vi "UI.vi"(0 "reference in":refnum<class "GUI Script Editor.lvclass">, 5 "error in (no error)":errorcluster) -> (14 "reference out":refnum<class "GUI Script Editor.lvclass">, 19 "error out":errorcluster)   [LabVIEW 2019, in "GUI Script Editor.lvclass"]
uses:
  GUI Script Editor.lvclass
  D:/H4000/src/GUI_class/GUI.lvclass
  TypeDef/GUI Step.ctl
  GUI_class/GUI.lvclass/GUI.ctl
  ConfigJSON_class/ConfigJSON.lvclass
  TypeDef/Script.ctl
  TypeDef/Step.ctl
  TypeDef/Direction.ctl
  ConfigJSON_class/ConfigJSON.lvclass/ConfigJSON.ctl
  99d7901a-116f-403a-a3f6-606aa629af4a.vi
  e526d8fc-7282-4644-9dda-8724ecf4fc0a.vi
  GUI_class/Set Win State.vi
  GUI_class/protected/GetSheredData.vi
  GUI_class/GUI.lvclass
  45f5d260-08a4-4eac-ba28-dc2dcf1a59bc.vi
  ConfigInterface_class/ConfigInterface.lvclass
  2ddd2a0d-c32e-4038-aee9-799db4cb2551.vi
panel:
  in  "GUI Step":T1
  in  "create":bool
  in  "Add Step":bool
  out "XY Graph - Dark":cluster{"X":dbl[], "Y":dbl[]}[](graph) caption="Давление"
  in  "Delete step":bool
  out "Program name":string="Название"
  in  "Save As":bool
  in  "Open":bool
  in  "Save":bool
  in  "Steps":i32(listbox)
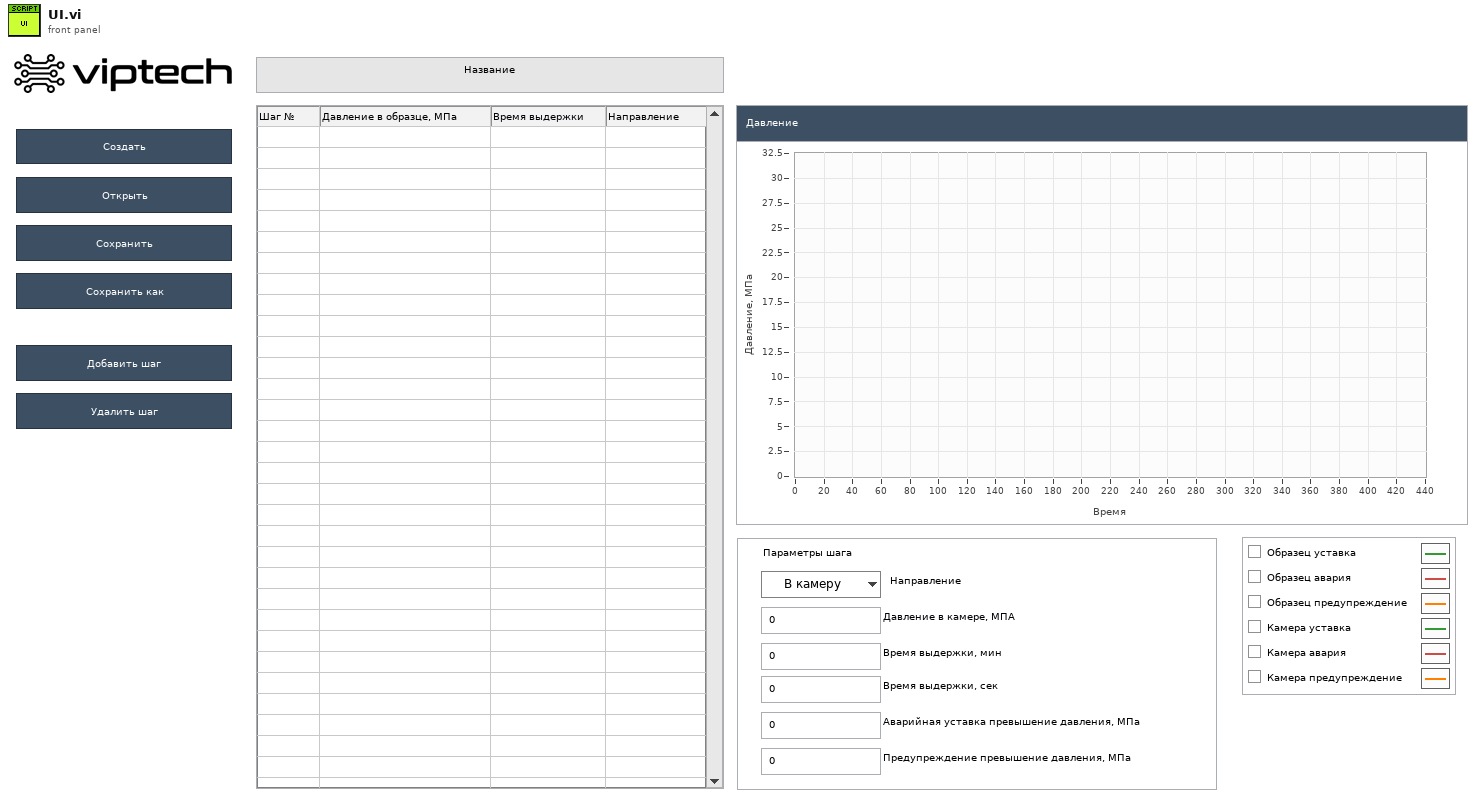
[diagram p1: front panel]
types:
  T1 = typedef "GUI Step.ctl" = cluster{"pressure MPa":dbl, "time min":dbl, "delta alarm MPa":dbl, "direction":enum16{"В камеру", "В образец"}, "delta warning MPa":dbl, "time sec":dbl}
  T2 = typedef "Script.ctl" = cluster{"Steps":T3[]}
  T3 = typedef "Step.ctl" = cluster{"Direction":T4, "Pressure MPa":dbl, "Time s":dbl, "Delta alarm MPa":dbl, "Delta warning MPa":dbl}
  T4 = typedef "Direction.ctl" = enum16{"Chamber", "DUT"}
  T5 = enum32{"Invalid", "Standard", "Closed", "Hidden", "Minimized", "Maximized"}
  T6 = enum32{"invalid app kind", "Development System", "Run Time System", "Student Edition", "Embedded LabVIEW", "Evaluation", "Custom"}
  T7 = cluster{"Core":cluster{"Current VI Reference":refnum<vi>, "Close Panel on Exit?":bool}, "Dir Scripts":path, "Curr Script":T2, "selected path":path, "Steps ref":refnum<vi>}
  T8 = cluster{"Current VI Reference":refnum<vi>, "Close Panel on Exit?":bool}
  T9 = typedef "GUI Paths.ctl" = cluster{"Dir Data":path, "Dir Setting":path, "SensorLib":path, "Dir Scripts":path}
  T10 = typedef "GUI Alarm customer settings.ctl" = cluster{"HIHI AI2":dbl, "HI AI2":dbl, "HIHI AI3":dbl, "HI AI3":dbl, "ENG0 OFF TIMEOUT":dbl, "ENG0 ON TIMEOUT":dbl, "HIHI AI7":dbl, "HI AI7":dbl, "HIHI AI6":dbl, "HI AI6":dbl, "HIHI AI5":dbl, "HI AI5":dbl}
  T11 = typedef "GUI Alarm developer settings.ctl" = cluster{"HIHI AI2":dbl, "HI AI2":dbl, "HIHI AI0":dbl, "HI AI0":dbl, "LOLO AI0":dbl, "LO AI0":dbl, "ENG2 OFF TIMEOUT":dbl, "ENG2 ON TIMEOUT":dbl, "HIHI AI3":dbl, "HI AI3":dbl, "HIHI AI1":dbl, "HI AI1":dbl, "LOLO AI1":dbl, "LO AI1":dbl, "ENG1 OFF TIMEOUT":dbl, "ENG1 ON TIMEOUT":dbl, "ENG0 OFF TIMEOUT":dbl, "ENG0 ON TIMEOUT":dbl, "LOLO AI8":dbl, "LO AI8":dbl, "LOLO AI9":dbl, "LO AI9":dbl, "LOLO AI5":dbl, "LO AI5":dbl, "Out Of Range HI":dbl, "Out Of Range LO":dbl}
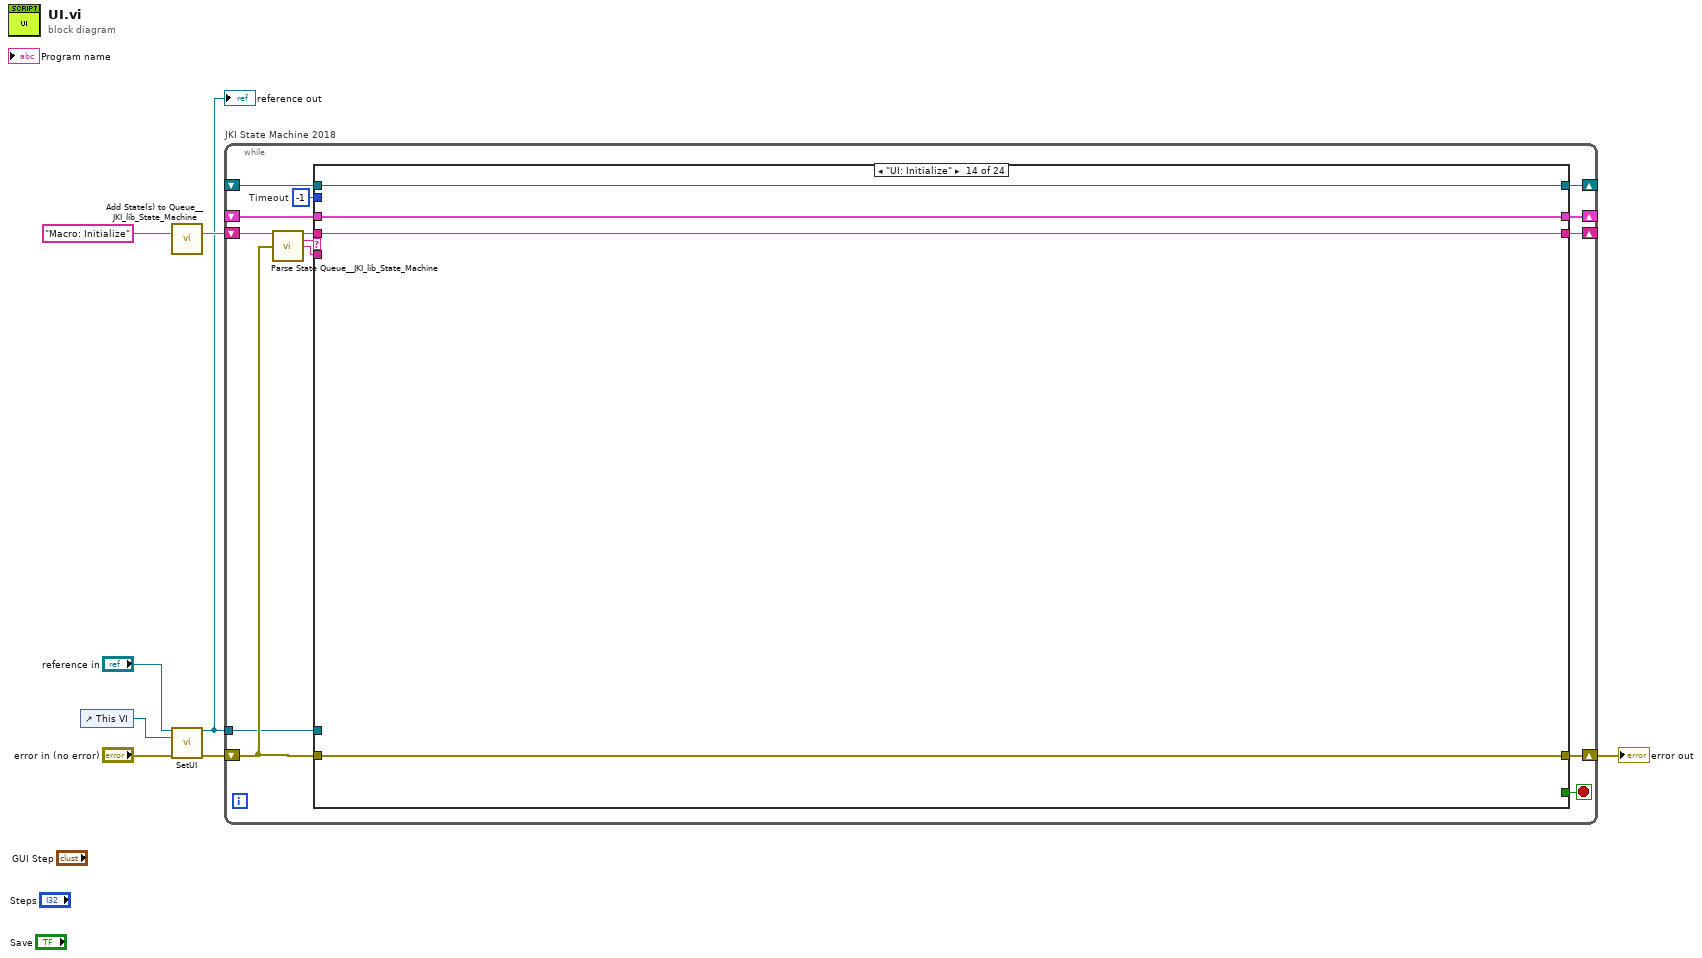
[diagram p0: block diagram]
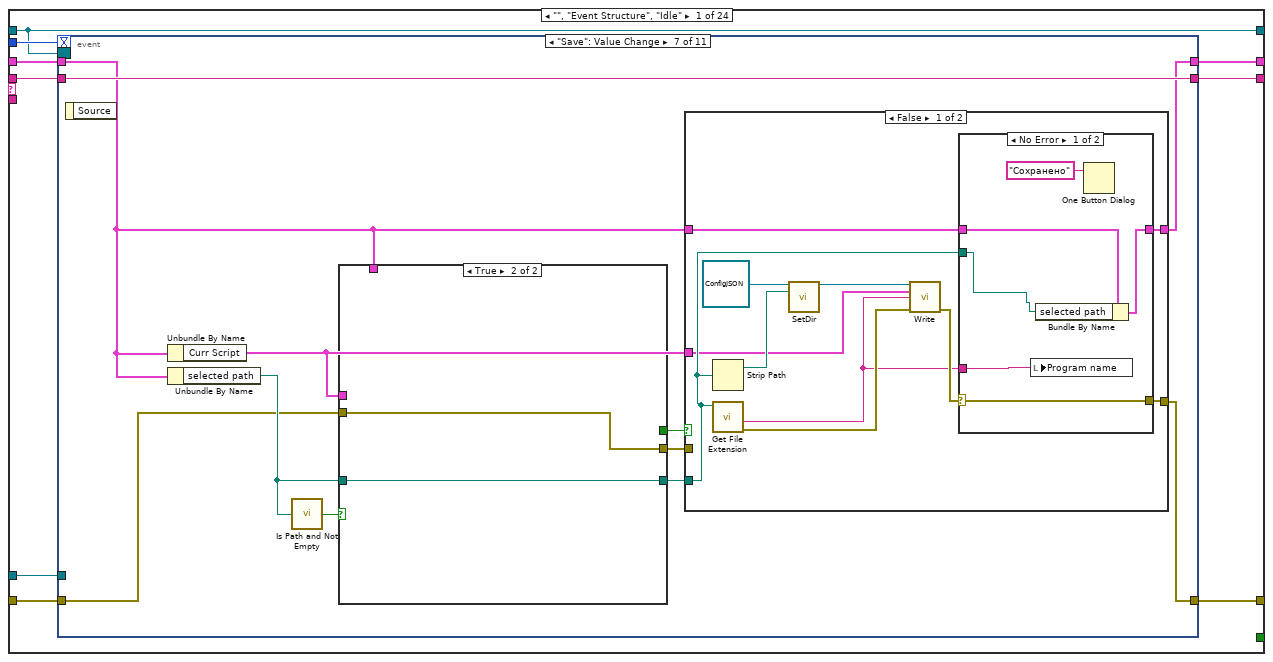
[diagram p2: hidden frame]
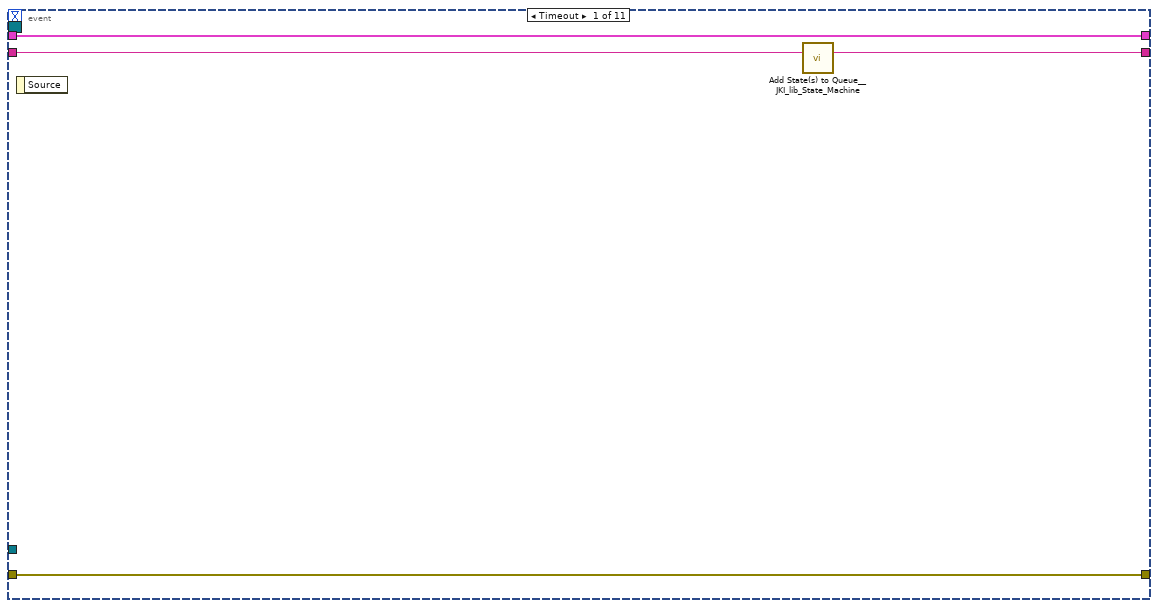
[diagram p3: hidden frame]
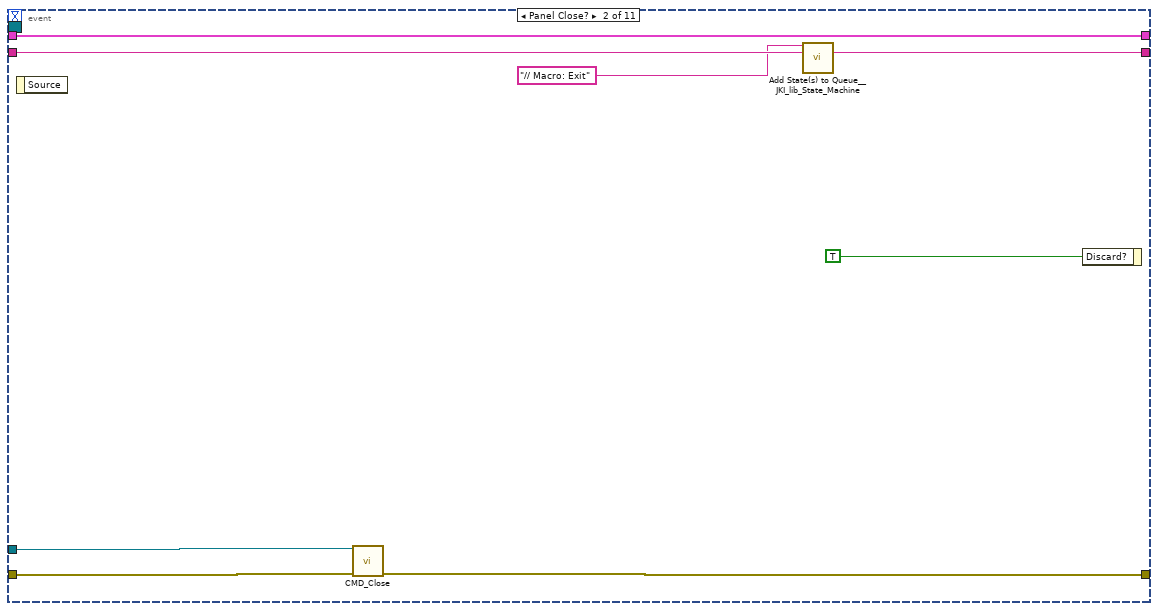
[diagram p4: hidden frame]
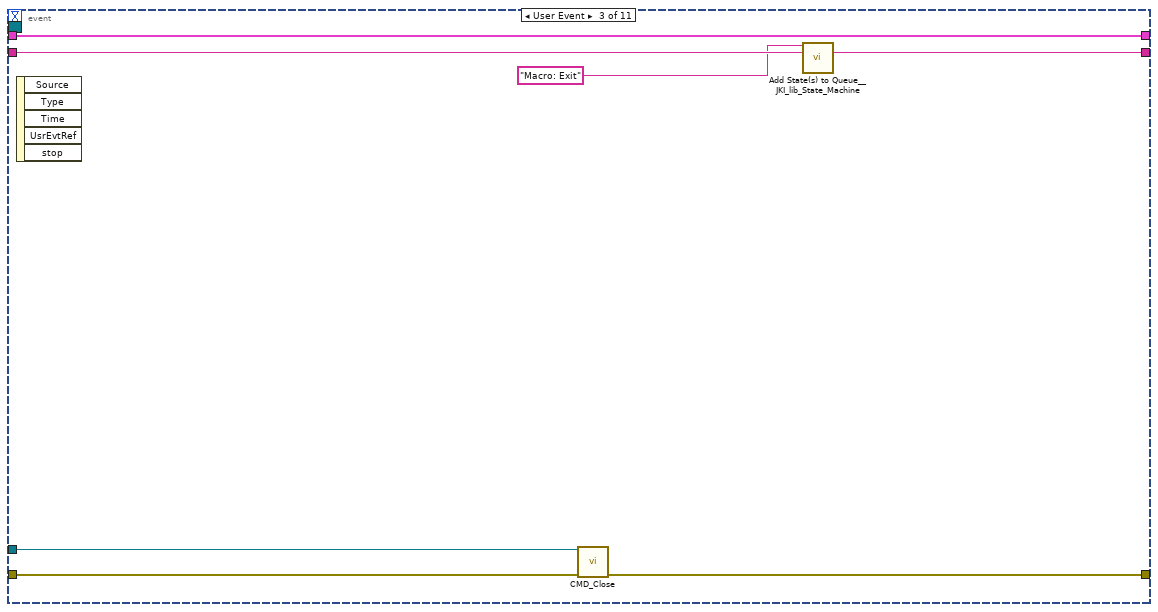
[diagram p5: hidden frame]
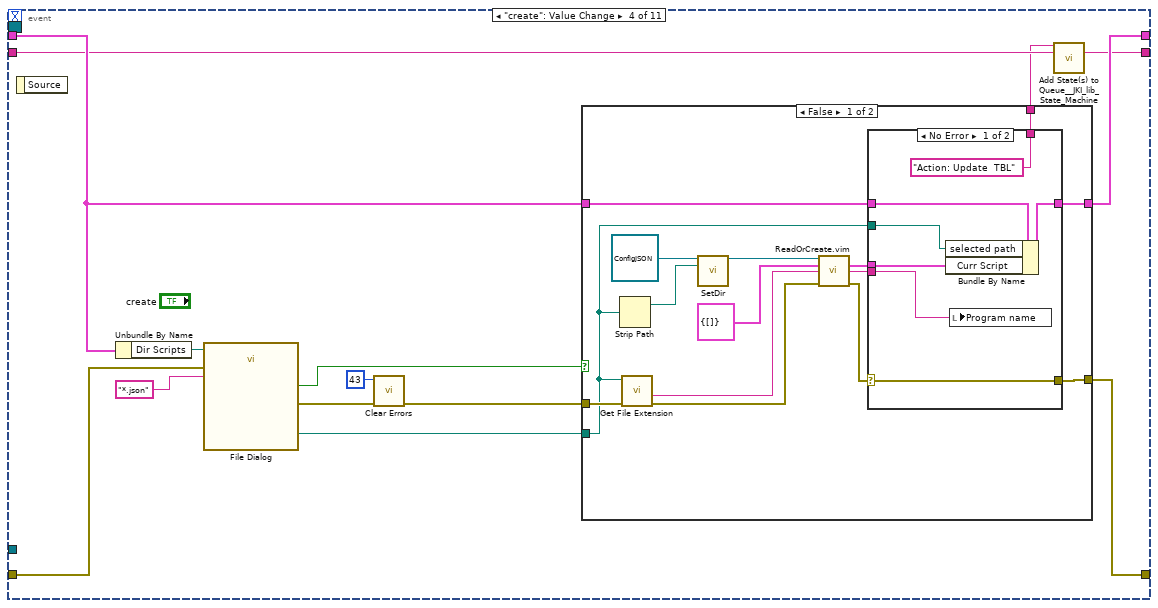
[diagram p6: hidden frame]
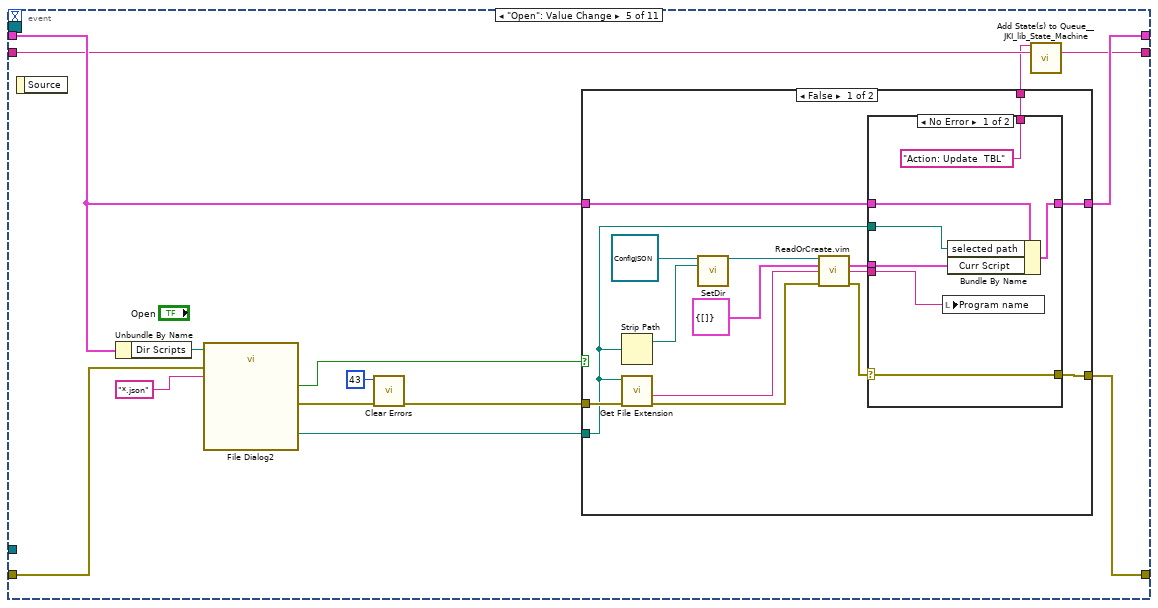
[diagram p9: hidden frame]
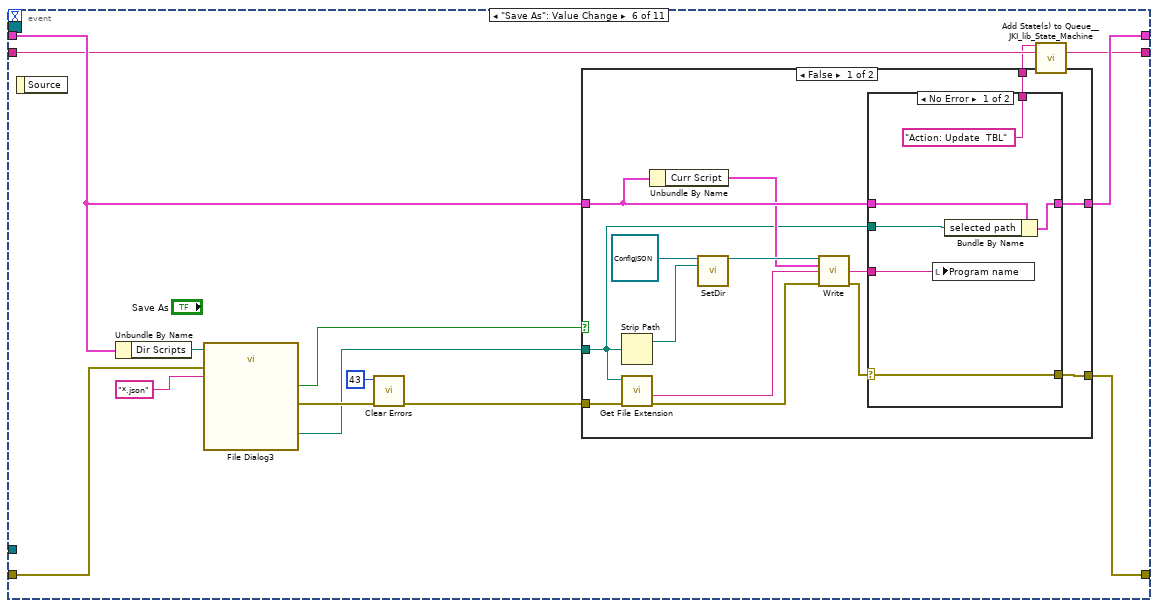
[diagram p12: hidden frame]
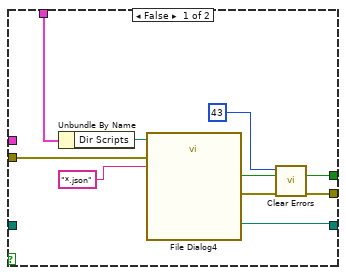
[diagram p17: hidden frame]
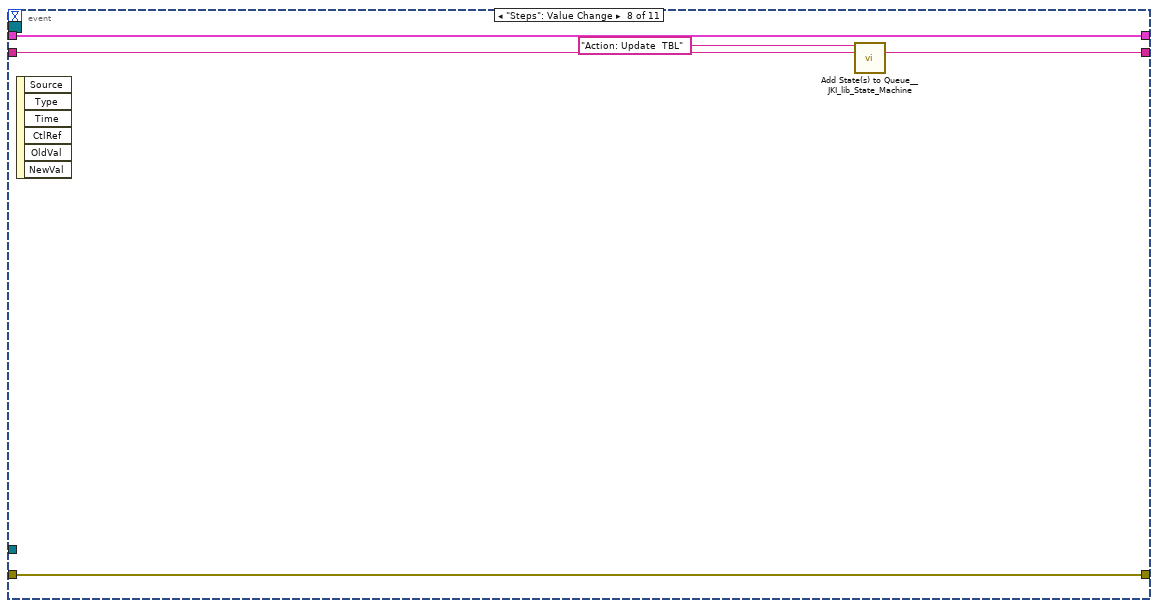
[diagram p18: hidden frame]
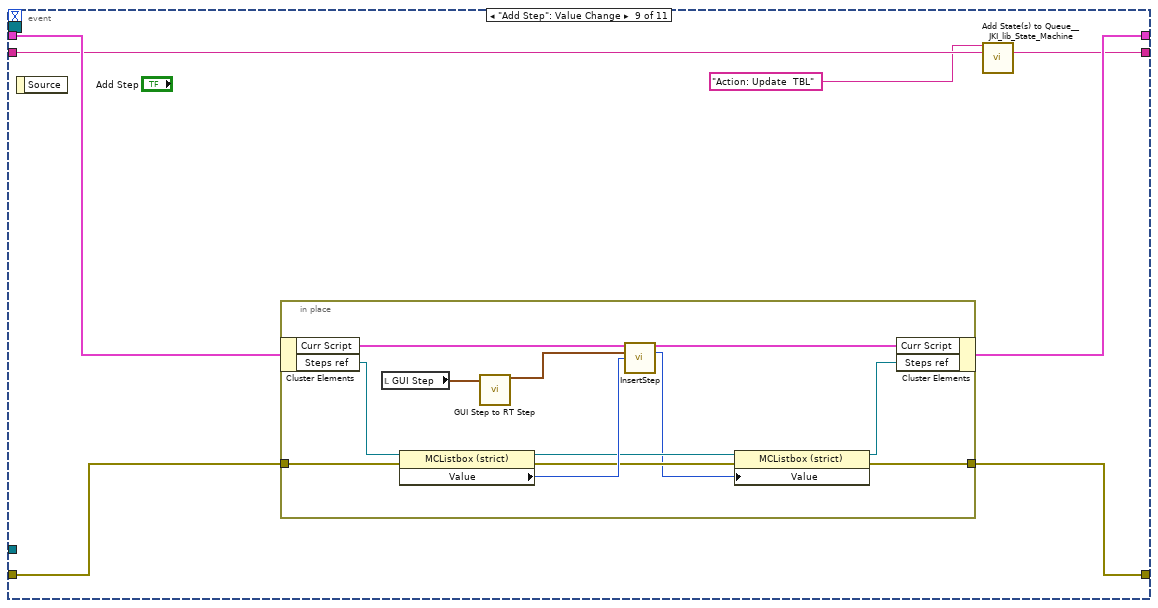
[diagram p19: hidden frame]
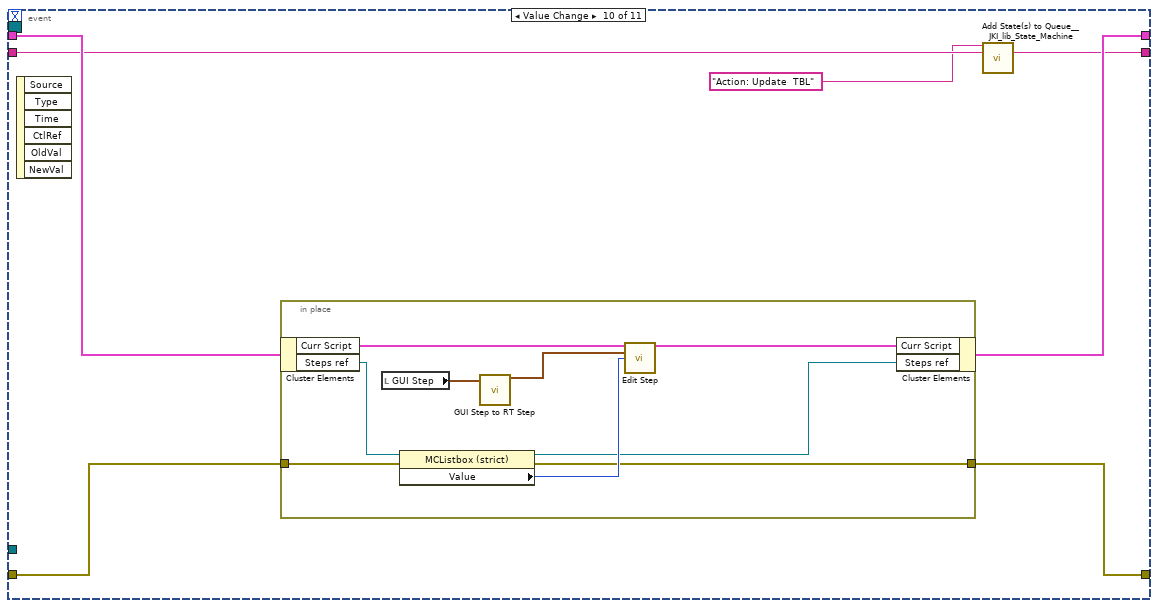
[diagram p20: hidden frame]
diagram:
  n1 = control-ref of="This VI"() -> (w3:refnum<vi>)
  n2 = call <vilib>:"Add State(s) to Queue__JKI_lib_State_Machine.vi"("State(s) in (\"\")"="Macro: Initialize") -> ("States Out"=w8:string)  [unwired: 14 in]
  n3 = call "SetUI.vi"("reference in"="reference in", "UI VI"=w3, "error in (no error)"="error in (no error)") -> ("reference out"=w1:refnum<class "GUI Script Editor.lvclass">, "error out"=w2:errorcluster)  [unwired: 11 in]
  "reference out" <- w1
  n4 = while "JKI State Machine 2018" {
    shift-right: [w15] -> _
    shift-left: _ -> [w14]
    shift-right: [w18] -> w6
    shift-left: w2 -> [w12]
    shift-right: [w17] -> _
    shift-left: w8 -> [w19]
    tunnel: w1 -> [w11]
    shift-right: [w10] -> _
    shift-left: _ -> [w9]
    stop <- w16 stop-if-true
    w13 = -1  # Timeout
    n5 = call <vilib>:"Parse State Queue__JKI_lib_State_Machine.vi"("State Queue"=w19, "Error In (no error)"=w12) -> ("Remaining States"=w21:string, "Current State"=w22:string, "Arguments"=w20:string)  [unwired: 11 in]
    n6 = case shown="\"UI: Initialize\"" w22 {
      selector: w22 -> [_ _ w275 _ _ _ _ _ _ _ _ _ _ _ _ _ _ _ _ _ _ _ _ _]
      tunnel: w21 -> [w31 w273 w279 w299 w306 w312 w317 w328 w335 w340 w347 w353 w358 w362 w369 w381 w451 w457 w463 w475 w479 w488 w512 w539]
      tunnel: w20 -> [_ _ _ _ _ _ _ _ _ _ _ _ _ _ w364 w375 _ _ _ _ _ _ _ _]
      tunnel: w14 -> [w29 w270 w277 w292 w303 w310 w314 _ w330 w337 w346 w351 w355 w361 w367 w377 w448 w454 w460 w472 w477 w483 w508 w538]
      tunnel: [w28 w271 w281 w296 errorcluster {"status"=FALSE, "code"=0, "source"=""} ("error out") w309 w315 w321 w331 w338 w344 w348 w356 w360 w365 w378 w449 w455 w461 w473 w478 w482 w507 w534] -> w18
      tunnel: w12 -> [w27 w271 w280 w296 w302 w309 w315 w323 w332 w338 w343 w349 w356 w360 w366 w379 w449 w455 w461 w473 w478 w481 w509 w535]
      tunnel: [w30 w272 w278 w298 w305 w311 w316 w328 w334 w339 w347 w352 w357 w362 w368 w380 w450 w456 w462 w474 w479 w488 w512 w539] -> w17
      tunnel: [_ _ _ _ _ TRUE _ _ _ _ _ _ _ _ _ _ _ _ _ _ _ _ _ _] -> w16
      tunnel: [w26 w270 w277 w297 w303 w310 w314 w327 w330 w337 w346 w351 w355 w361 w367 w377 w448 w454 w460 w472 w477 w486 w508 w538] -> w15
      tunnel: w13 -> [w25 _ _ _ _ _ _ _ _ _ _ _ _ _ _ _ _ _ _ _ _ _ _ _]
      tunnel: w11 -> [w24 _ _ _ _ _ _ _ _ _ w342 _ _ _ _ _ _ _ _ _ _ w485 w510 _]
      tunnel: [w23 w269 w274 w286 w300 w307 w313 w325 w329 w336 w345 w350 w354 w359 w363 w374 w447 w452 w458 w465 w476 w487 w511 w540] -> w10
      tunnel: w9 -> [w23 w269 w274 w286 w300 w307 w313 w325 w329 w336 _ w350 w354 w359 w363 w374 w447 w452 w458 w465 w476 w487 w511 w540]
      frame "", "Event Structure", "Idle" {
        n7 = event shown="[6] \"Save\": Value Change" {
          selector: w23 -> [_ _ _ _ _ _ _ _ _ _ _]
          dyn-events: _ -> [_ _ _ _ _ _ _ _ _ _ _]
          timeout: w25 -> [_ _ _ _ _ _ _ _ _ _ _]
          tunnel: w31 -> [w35 w43 w50 w52 w92 w132 w179 w213 w218 w237 w253]
          tunnel: [w34 w42 w49 w53 w93 w133 w179 w214 w219 w238 w254] -> w30
          tunnel: w29 -> [w32 w41 w48 w55 w95 w135 w171 w215 w223 w242 w258]
          tunnel: [w33 w36 w44 w57 w97 w137 w178 w216 w220 w239 w255] -> w28
          tunnel: w27 -> [w33 w37 w45 w63 w103 w143 w173 w216 w221 w240 w256]
          tunnel: [w32 w41 w48 w54 w94 w134 w177 w215 w222 w241 w257] -> w26
          tunnel: w24 -> [_ w38 w46 _ _ _ _ _ _ _ _]
          event Timeout {
            n8 = event-data() -> ()  [unwired: 1 in, 1 out]
            n9 = call <vilib>:"Add State(s) to Queue__JKI_lib_State_Machine.vi"("State(s) in (\"\")"=w35) -> ("States Out"=w34:string)  [unwired: 14 in]
          }
          event Panel Close? {
            n10 = event-data() -> ()  [unwired: 1 in, 1 out]
            n11 = call "CMD_Close.vi"("reference in"=w38, "error in (no error)"=w37) -> ("error out"=w36:errorcluster)  [unwired: 12 in, 1 out]
            n12 = call <vilib>:"Add State(s) to Queue__JKI_lib_State_Machine.vi"("State(s) in Front (\"\")"="// Macro: Exit", "State(s) in (\"\")"=w43) -> ("States Out"=w42:string)  [unwired: 13 in]
            n13 = event-data("Discard?"=TRUE) -> ()  [unwired: 1 in, 1 out]
          }
          event User Event {
            n14 = event-data() -> ()  [unwired: 1 in, 5 out]
            n15 = call "CMD_Close.vi"("reference in"=w46, "error in (no error)"=w45) -> ("error out"=w44:errorcluster)  [unwired: 12 in, 1 out]
            n16 = call <vilib>:"Add State(s) to Queue__JKI_lib_State_Machine.vi"("State(s) in Front (\"\")"="Macro: Exit", "State(s) in (\"\")"=w50) -> ("States Out"=w49:string)  [unwired: 13 in]
          }
          event "create": Value Change {
            n17 = event-data() -> ()  [unwired: 1 in, 1 out]
            n18 = Unbundle By Name(w55) -> ("Dir Scripts"=w64:path)
            n19 = call "File Dialog"("start path"=w64, "error in"=w63, "pattern (all files)"="*.json") -> ("selected path"=w56:path, "cancelled"=w58:bool, "error out"=w60:errorcluster)  [unwired: 9 in, 1 out]
            n20 = call <vilib>:"Clear Errors.vi"("error in (no error)"=w60, "specific error code to clear (0: all)"=43) -> ("error out"=w59:errorcluster)  [unwired: 4 in, 1 out]
            n21 = case shown="False" w58 {
              tunnel: w59 -> [w76 w90]
              tunnel: [w71 w90] -> w57
              tunnel: w56 -> [w66 _]
              tunnel: w55 -> [w70 w89]
              tunnel: [w69 w89] -> w54
              tunnel: [w65 _] -> w51
              frame False {
                n22 = Strip Path(path=w66) -> (stripped path=w77:path)  [unwired: 1 out]
                n23 = call <vilib>:"Get File Extension.vi"("error in (no error)"=w76, "file"=w66) -> ("error out"=w73:errorcluster, "filename without extension"=w75:string)  [unwired: 5 in, 3 out]
                n24 = call "SetDir.vi"("reference in"=refnum<class "ConfigJSON.lvclass"> refnum ("ConfigJSON"), "Config Dir"=w77) -> ("JSON"=w78:refnum<class "ConfigJSON.lvclass">)  [unwired: 13 in]
                n25 = call "ReadOrCreate.vim"("reference in"=w78, "Type and Defaults"=T2 {"Steps"=[]} ("Script"), "Name"=w75, "error in (no error)"=w73) -> ("Data"=w68:T2, "Name dub"=w67:string, "error out"=w72:errorcluster)  [unwired: 7 in, 2 out]
                n26 = case shown="No Error" w72 {
                  selector: w72 -> [w83 w88]
                  tunnel: [w83 w88] -> w71
                  tunnel: w70 -> [w86 w87]
                  tunnel: [w85 w87] -> w69
                  tunnel: w68 -> [w84 _]
                  tunnel: w67 -> [w82 _]
                  tunnel: w66 -> [w81 _]
                  tunnel: ["Action: Update  TBL" ("State(s) in Front (\"\")") _] -> w65
                  frame No Error {
                    n27 = Bundle By Name(cluster=w86, "selected path"=w81, "Curr Script"=w84) -> (w85:T7)
                    n28 = local write "Program name"(w82) -> ()
                  }
                  frame Error {
                  }
                }
              }
              frame True {
              }
            }
            n29 = call <vilib>:"Add State(s) to Queue__JKI_lib_State_Machine.vi"("State(s) in Front (\"\")"=w51, "State(s) in (\"\")"=w52) -> ("States Out"=w53:string)  [unwired: 13 in]
          }
          event "Open": Value Change {
            n30 = event-data() -> ()  [unwired: 1 in, 1 out]
            n31 = Unbundle By Name(w95) -> ("Dir Scripts"=w104:path)
            n32 = call "File Dialog2"("start path"=w104, "error in"=w103, "pattern (all files)"="*.json") -> ("selected path"=w96:path, "cancelled"=w98:bool, "error out"=w100:errorcluster)  [unwired: 9 in, 1 out]
            n33 = call <vilib>:"Clear Errors.vi"("error in (no error)"=w100, "specific error code to clear (0: all)"=43) -> ("error out"=w99:errorcluster)  [unwired: 4 in, 1 out]
            n34 = case shown="False" w98 {
              tunnel: w99 -> [w116 w130]
              tunnel: [w111 w130] -> w97
              tunnel: w96 -> [w106 _]
              tunnel: w95 -> [w110 w129]
              tunnel: [w109 w129] -> w94
              tunnel: [w105 _] -> w91
              frame False {
                n35 = Strip Path(path=w106) -> (stripped path=w117:path)  [unwired: 1 out]
                n36 = call <vilib>:"Get File Extension.vi"("error in (no error)"=w116, "file"=w106) -> ("error out"=w113:errorcluster, "filename without extension"=w115:string)  [unwired: 5 in, 3 out]
                n37 = call "SetDir.vi"("reference in"=refnum<class "ConfigJSON.lvclass"> refnum ("ConfigJSON"), "Config Dir"=w117) -> ("JSON"=w118:refnum<class "ConfigJSON.lvclass">)  [unwired: 13 in]
                n38 = call "ReadOrCreate.vim"("reference in"=w118, "Type and Defaults"=T2 {"Steps"=[]} ("Script"), "Name"=w115, "error in (no error)"=w113) -> ("Data"=w108:T2, "Name dub"=w107:string, "error out"=w112:errorcluster)  [unwired: 7 in, 2 out]
                n39 = case shown="No Error" w112 {
                  selector: w112 -> [w123 w128]
                  tunnel: [w123 w128] -> w111
                  tunnel: w110 -> [w126 w127]
                  tunnel: [w125 w127] -> w109
                  tunnel: w108 -> [w124 _]
                  tunnel: w107 -> [w122 _]
                  tunnel: w106 -> [w121 _]
                  tunnel: ["Action: Update  TBL" ("State(s) in Front (\"\")") _] -> w105
                  frame No Error {
                    n40 = local write "Program name"(w122) -> ()
                    n41 = Bundle By Name(cluster=w126, "selected path"=w121, "Curr Script"=w124) -> (w125:T7)
                  }
                  frame Error {
                  }
                }
              }
              frame True {
              }
            }
            n42 = call <vilib>:"Add State(s) to Queue__JKI_lib_State_Machine.vi"("State(s) in Front (\"\")"=w91, "State(s) in (\"\")"=w92) -> ("States Out"=w93:string)  [unwired: 13 in]
          }
          event "Save As": Value Change {
            n43 = event-data() -> ()  [unwired: 1 in, 1 out]
            n44 = Unbundle By Name(w135) -> ("Dir Scripts"=w144:path)
            n45 = call "File Dialog3"("start path"=w144, "error in"=w143, "pattern (all files)"="*.json") -> ("selected path"=w136:path, "cancelled"=w138:bool, "error out"=w140:errorcluster)  [unwired: 9 in, 1 out]
            n46 = call <vilib>:"Clear Errors.vi"("error in (no error)"=w140, "specific error code to clear (0: all)"=43) -> ("error out"=w139:errorcluster)  [unwired: 4 in, 1 out]
            n47 = case shown="False" w138 {
              tunnel: w139 -> [w155 w168]
              tunnel: [w151 w168] -> w137
              tunnel: w136 -> [w146 _]
              tunnel: w135 -> [w148 w167]
              tunnel: [w150 w167] -> w134
              tunnel: [w145 _] -> w131
              frame False {
                n48 = Strip Path(path=w146) -> (stripped path=w156:path)  [unwired: 1 out]
                n49 = call <vilib>:"Get File Extension.vi"("error in (no error)"=w155, "file"=w146) -> ("error out"=w153:errorcluster, "filename without extension"=w154:string)  [unwired: 5 in, 3 out]
                n50 = Unbundle By Name(w148) -> ("Curr Script"=w147:T2)
                n51 = call "SetDir.vi"("reference in"=refnum<class "ConfigJSON.lvclass"> refnum ("ConfigJSON"), "Config Dir"=w156) -> ("JSON"=w157:refnum<class "ConfigJSON.lvclass">)  [unwired: 13 in]
                n52 = call-dynamic "Write.vi"("reference in"=w157, "Data"=w147, "Name"=w154, "error in (no error)"=w153) -> ("Name dub"=w149:string, "error out"=w152:errorcluster)  [unwired: 8 in, 2 out]
                n53 = case shown="No Error" w152 {
                  selector: w152 -> [w162 w166]
                  tunnel: [w162 w166] -> w151
                  tunnel: w148 -> [w164 w165]
                  tunnel: [w163 w165] -> w150
                  tunnel: w149 -> [w161 _]
                  tunnel: w146 -> [w160 _]
                  tunnel: ["Action: Update  TBL" ("State(s) in Front (\"\")") _] -> w145
                  frame No Error {
                    n54 = local write "Program name"(w161) -> ()
                    n55 = Bundle By Name(cluster=w164, "selected path"=w160) -> (w163:T7)
                  }
                  frame Error {
                  }
                }
              }
              frame True {
              }
            }
            n56 = call <vilib>:"Add State(s) to Queue__JKI_lib_State_Machine.vi"("State(s) in Front (\"\")"=w131, "State(s) in (\"\")"=w132) -> ("States Out"=w133:string)  [unwired: 13 in]
          }
          event "Save": Value Change {
            n57 = event-data() -> ()  [unwired: 1 in, 1 out]
            n58 = Unbundle By Name(w171) -> ("Curr Script"=w172:T2)
            n59 = Unbundle By Name(w171) -> ("selected path"=w174:path)
            n60 = call <vilib>:"Is Path and Not Empty.vi"("path"=w174) -> ("Is Path and Not Empty?"=w176:bool)  [unwired: 4 in]
            n61 = case shown="True" w176 {
              tunnel: [w206 w211] -> w175
              tunnel: w174 -> [_ w211]
              tunnel: w173 -> [w207 w210]
              tunnel: w172 -> [_ _]
              tunnel: w171 -> [w205 _]
              tunnel: [w204 _] -> w170
              tunnel: [w201 w210] -> w169
              frame False {
                n62 = Unbundle By Name(w205) -> ("Dir Scripts"=w209:path)
                n63 = call "File Dialog4"("start path"=w209, "error in"=w207, "pattern (all files)"="*.json") -> ("selected path"=w206:path, "cancelled"=w204:bool, "error out"=w202:errorcluster)  [unwired: 9 in, 1 out]
                n64 = call <vilib>:"Clear Errors.vi"("error in (no error)"=w202, "specific error code to clear (0: all)"=43) -> ("error out"=w201:errorcluster)  [unwired: 4 in, 1 out]
              }
              frame True {
              }
            }
            n65 = case shown="False" w170 {
              tunnel: [w190 w199] -> w178
              tunnel: [w189 w200] -> w177
              tunnel: w175 -> [w183 _]
              tunnel: w172 -> [w182 _]
              tunnel: w171 -> [w181 w200]
              tunnel: w169 -> [_ w199]
              frame False {
                n66 = Strip Path(path=w183) -> (stripped path=w186:path)  [unwired: 1 out]
                n67 = call <vilib>:"Get File Extension.vi"("file"=w183) -> ("error out"=w185:errorcluster, "filename without extension"=w180:string)  [unwired: 6 in, 3 out]
                n68 = call "SetDir.vi"("reference in"=refnum<class "ConfigJSON.lvclass"> refnum ("ConfigJSON"), "Config Dir"=w186) -> ("JSON"=w187:refnum<class "ConfigJSON.lvclass">)  [unwired: 13 in]
                n69 = call-dynamic "Write.vi"("reference in"=w187, "Data"=w182, "Name"=w180, "error in (no error)"=w185) -> ("error out"=w184:errorcluster)  [unwired: 8 in, 3 out]
                n70 = case shown="No Error" w184 {
                  selector: w184 -> [w196 w198]
                  tunnel: [w196 w198] -> w190
                  tunnel: w181 -> [w192 w197]
                  tunnel: [w191 w197] -> w189
                  tunnel: w183 -> [w193 _]
                  tunnel: w180 -> [w194 _]
                  frame No Error {
                    n71 = local write "Program name"(w194) -> ()
                    n72 = Bundle By Name(cluster=w192, "selected path"=w193) -> (w191:T7)
                    n73 = One Button Dialog(message="Сохранено") -> ()  [unwired: 1 in, 1 out]
                  }
                  frame Error {
                  }
                }
              }
              frame True {
              }
            }
          }
          event "Steps": Value Change {
            n74 = event-data() -> ()  [unwired: 1 in, 6 out]
            n75 = call <vilib>:"Add State(s) to Queue__JKI_lib_State_Machine.vi"("State(s) in Front (\"\")"="Action: Update  TBL" ("State(s) in Front (\"\")"), "State(s) in (\"\")"=w213) -> ("States Out"=w214:string)  [unwired: 13 in]
          }
          event "Add Step": Value Change {
            n76 = event-data() -> ()  [unwired: 1 in, 1 out]
            n77 = in-place {
              in-place-border: w221 -> [w229]
              in-place-border: [w225] -> w220
              n78 = in-place-cluster #1(w223) -> ("Curr Script"=w235:T2, "Steps ref"=w232:refnum<vi>)
              n79 = local read "GUI Step"() -> (w231:T1)
              n80 = property class="MCListbox (strict)"(reference=w232, error in=w229) -> (reference out=w227:refnum<vi>, error out=w228:errorcluster, "Value"=w233:i32)
              n81 = call "GUI Step to RT Step.vi"("GUI Step"=w231) -> ("STEP"=w230:T3)  [unwired: 14 in]
              n82 = call "InsertStep.vi"("Script in"=w235, "new element/subarray"=w230, "index in"=w233) -> ("Script out"=w234:T2, "index out"=w224:i32)  [unwired: 11 in]
              n83 = property class="MCListbox (strict)"(reference=w227, error in=w228, "Value"=w224) -> (reference out=w226:refnum<vi>, error out=w225:errorcluster)
              n84 = in-place-cluster #1("Curr Script"=w234, "Steps ref"=w226) -> (w222:T7)
            }
            n85 = call <vilib>:"Add State(s) to Queue__JKI_lib_State_Machine.vi"("State(s) in Front (\"\")"="Action: Update  TBL" ("State(s) in Front (\"\")"), "State(s) in (\"\")"=w218) -> ("States Out"=w219:string)  [unwired: 13 in]
          }
          event Value Change {
            n86 = event-data() -> ()  [unwired: 1 in, 6 out]
            n87 = in-place {
              in-place-border: w240 -> [w245]
              in-place-border: [w244] -> w239
              n88 = in-place-cluster #2(w242) -> ("Curr Script"=w251:T2, "Steps ref"=w248:refnum<vi>)
              n89 = local read "GUI Step"() -> (w247:T1)
              n90 = property class="MCListbox (strict)"(reference=w248, error in=w245) -> (reference out=w243:refnum<vi>, error out=w244:errorcluster, "Value"=w249:i32)
              n91 = call "GUI Step to RT Step.vi"("GUI Step"=w247) -> ("STEP"=w246:T3)  [unwired: 14 in]
              n92 = call "Edit Step.vi"("Script in"=w251, "new element/subarray"=w246, "index"=w249) -> ("Script out"=w250:T2)  [unwired: 12 in]
              n93 = in-place-cluster #2("Curr Script"=w250, "Steps ref"=w243) -> (w241:T7)
            }
            n94 = call <vilib>:"Add State(s) to Queue__JKI_lib_State_Machine.vi"("State(s) in Front (\"\")"="Action: Update  TBL" ("State(s) in Front (\"\")"), "State(s) in (\"\")"=w237) -> ("States Out"=w238:string)  [unwired: 13 in]
          }
          event "Delete step": Value Change {
            n95 = event-data() -> ()  [unwired: 1 in, 6 out]
            n96 = in-place {
              in-place-border: w256 -> [w264]
              in-place-border: [w261] -> w255
              n97 = in-place-cluster #3(w258) -> ("Curr Script"=w268:T2, "Steps ref"=w265:refnum<vi>)
              n98 = property class="MCListbox (strict)"(reference=w265, error in=w264) -> (reference out=w263:refnum<vi>, error out=w262:errorcluster, "Value"=w266:i32)
              n99 = call "deleteStep.vi"("Script in"=w268, "index in"=w266) -> ("Script out"=w267:T2, "index out"=w259:i32)  [unwired: 12 in]
              n100 = property class="MCListbox (strict)"(reference=w263, error in=w262, "Value"=w259) -> (reference out=w260:refnum<vi>, error out=w261:errorcluster)
              n101 = in-place-cluster #3("Curr Script"=w267, "Steps ref"=w260) -> (w257:T7)
            }
            n102 = call <vilib>:"Add State(s) to Queue__JKI_lib_State_Machine.vi"("State(s) in Front (\"\")"="Action: Update  TBL" ("State(s) in Front (\"\")"), "State(s) in (\"\")"=w253) -> ("States Out"=w254:string)  [unwired: 13 in]
          }
        }
      }
      frame "---------- Core ----------" {
        n103 = call <vilib>:"Add State(s) to Queue__JKI_lib_State_Machine.vi"("State(s) in (\"\")"=w273) -> ("States Out"=w272:string)  [unwired: 14 in]
      }
      frame Default {
        w284 = 42 items=["No error", "Argument error", "Memory is full", "Out of zone", "End of file", "File already open", "Generic file I/O error", "File not found", "File permission error", "Disk is full", "Duplicate path", "Too many files open", "System feature not enabled", "Resource file not found", "Cannot add resource", "Resource not found", "Image not found", "Image memory error", "Pen does not exist", "Config type invalid", "Config token not found", "Config parse error", "Config memory error", "Bad external code format", "Bad external code offset", "External code not present", "Null window", "Destroy window error", "Null menu", "Print aborted", "Bad print record", "Print driver error", "Windows error during printing", "Memory error during printing", "Print dialog error", "Generic print error", "Invalid device refnum", "Device not found", "Device parameter error", "Device unit error", "Cannot open device", "Device call aborted", "Generic error", "Cancelled by user", "Object ID too low", "Object ID too high", "Object not in heap", "Unknown heap", "Unknown object (invalid DefProc)", "Unknown object (DefProc not in table)", "Message out of range", "Invalid (null) method", "Unknown message", "Manager call not supported", "Bad address", "Network operation in progress", "Network operation timed out", "Connection is busy", "Network attribute not supported", "Network error", "Address in use", "System out of memory", "Connection aborted", "Connection refused", "Not connected", "Already connected", "Connection closed", "Initialization error (interapplication manager)", "Bad occurrence", "Wait on unbound occurrence handler", "Occurrence queue overflow", "Datalog type conflict", "Unused", "Unrecognized type (interapplication manager)", "Memory corrupt", "Failed to make temporary DLL", "Old CIN version", "Drag socket not found", "Failed to load drop-object", "Failed to register OLE object", "Failed to release OLE object", "Format specifier type mismatch", "Unknown format specifier", "Too few format specifiers", "Too many format specifiers", "Scan failed", "Newer CIN version", "Error converting to variant", "Runtime menu error", "Password tampered", "Variant attribute not found", "Incompatible variant data type", "Event data is not available", "Event Store is not present", "Occurrence is not found", "Event Queue is not created", "Event info is not available", "Refnum passed is NULL", "Error retrieving Class GUID", "Error retrieving CoClass GUID", "Error retrieving TypeLib GUID.", "Bad built application magic bytes.", "Specific driver is different from the specific driver associated with the Logical Name.", "There is no session opened to the class driver.", "Max Error", "MAX - Error with config objects", "MAX - Error loading configuration", "MAX - Group not supported"]
        # "Current State"
        # "Do not delete, rename, or modify this frame.\n(this is used to capture unhandled states and typos)"
        # "Handle mistyped state name (developer tool)"
        n104 = Format Into String(format string="Software Exception: Unhandled State \"%s\"." ("message"), error in=w280, w275) -> (resulting string=w283:string, error out=w282:errorcluster)  [unwired: 1 in]
        n105 = call <vilib>:"Error Cluster From Error Code.vi"("show call chain? (False)"=TRUE, "error in (no error)"=w282, "error message (\"\")"=w283, "error code (0)"=w284) -> ("error out"=w281:errorcluster)  [unwired: 5 in]
        n106 = call <vilib>:"Add State(s) to Queue__JKI_lib_State_Machine.vi"("State(s) in (\"\")"=w279) -> ("States Out"=w278:string)  [unwired: 14 in]
      }
      frame "Initialize Core Data" {
        # "Do not delete, rename, or modify this frame.\n(this is used to determine panel behavior on exit)"
        # "originally closed?"
        # "exe?"
        # "If panel starts closed or is an EXE, then close it when we exit"
        n107 = property class="VI"() -> ("FP.State"=w289:T5)  [unwired: 2 in, 2 out]
        n108 = property class="App"() -> ("App.Kind"=w295:T6)  [unwired: 2 in, 2 out]
        n109 = control-ref of="Current VI Reference"() -> (w290:refnum<vi>)
        n110 = Equal?(x=w289, y=T5."Closed" ("Front Panel Window:State")) -> (x = y?=w287:bool)
        n111 = Equal?(x=w295, y=T6."Run Time System" ("Application:Kind")) -> (x = y?=w293:bool)
        n112 = Or(x=w287, y=w293) -> (x .or. y?=w291:bool)
        n113 = Bundle By Name(cluster=w292, "Core.Current VI Reference"=w290, "Core.Close Panel on Exit?"=w291) -> (w297:T7)
        n114 = call <vilib>:"Add State(s) to Queue__JKI_lib_State_Machine.vi"("State(s) in (\"\")"=w299) -> ("States Out"=w298:string)  [unwired: 14 in]
      }
      frame "Error Handler" {
        # "Unhandled Error -- Display it"
        # "Handle any errors here.\nYou can also output any states to clean-up after errors occur"
        # "Clear error"
        n115 = call <vilib>:"General Error Handler.vi"("error in (no error)"=w302) -> ()  [unwired: 10 in, 5 out]
        n116 = call <vilib>:"Add State(s) to Queue__JKI_lib_State_Machine.vi"("State(s) in Front (\"\")"="/* Post Error States", "State(s) in (\"\")"=w306) -> ("States Out"=w305:string)  [unwired: 13 in]
      }
      frame "Exit" {
        # "Do not put any code in this frame.\n(No errors that occur here will be handled.)"
        n117 = call <vilib>:"Add State(s) to Queue__JKI_lib_State_Machine.vi"("State(s) in (\"\")"=w312) -> ("States Out"=w311:string)  [unwired: 14 in]
      }
      frame "---------- Data ----------" {
        # "Do not put any code in this frame.\n(It is a separator no-op. You can make a copy of this frame to create a new Data frame)"
        n118 = call <vilib>:"Add State(s) to Queue__JKI_lib_State_Machine.vi"("State(s) in (\"\")"=w317) -> ("States Out"=w316:string)  [unwired: 14 in]
      }
      frame "Data: Initialize" {
        w319 = path ""  # selected path
        w320 = T2 {"Steps"=[]}  # Curr Script
        w326 = T8 {"Current VI Reference"=refnum, "Close Panel on Exit?"=FALSE}  # Core
        n119 = call "GUI Get Paths.vi"("error in (no error)"=w323) -> ("Paths"=w324:T9, "error out"=w321:errorcluster)  [unwired: 13 in]
        n120 = Unbundle By Name(w324) -> ("Dir Scripts"=w322:path)
        n121 = control-ref of="Steps ref"() -> (w318:refnum<vi>)
        n122 = Bundle("Core"=w326, "Dir Scripts"=w322, "Curr Script"=w320, "selected path"=w319, "Steps ref"=w318) -> (w327:T7)  [unwired: 1 in]
      }
      frame "Data: Cleanup" {
        # "Cleanup any data and references, here.\n(this is called automatically, by the Macro: Exit)"
        n123 = Unbundle By Name(w330) -> ("Core.Current VI Reference"=w333:refnum<vi>)
        n124 = Close Reference(reference=w333, error in (no error)=w332) -> (error out=w331:errorcluster)
        n125 = call <vilib>:"Add State(s) to Queue__JKI_lib_State_Machine.vi"("State(s) in (\"\")"=w335) -> ("States Out"=w334:string)  [unwired: 14 in]
      }
      frame "---------- Events ----------" {
        # "Do not put any code in this frame.\n(It is a separator no-op. You can make a copy of this frame to create a new UI frame)"
        n126 = call <vilib>:"Add State(s) to Queue__JKI_lib_State_Machine.vi"("State(s) in (\"\")"=w340) -> ("States Out"=w339:string)  [unwired: 14 in]
      }
      frame "Events: Register" {
        n127 = call "Read stop event.vi"("GUI in"=w342) -> ("stop event"=w341:refnum<user-event>)  [unwired: 8 in, 2 out]
        n128 = register-events(error in=w343, w341) -> (reference out=w345:refnum<event-registration>, error out=w344:errorcluster)  [unwired: 1 in]
      }
      frame "Events: Unregister" {
        # "Do not put any code in this frame.\n(It is a separator no-op. You can make a copy of this frame to create a new UI frame)"
        n129 = Unregister For Events(event registration refnum=w350, error in=w349) -> (error out=w348:errorcluster)
        n130 = call <vilib>:"Add State(s) to Queue__JKI_lib_State_Machine.vi"("State(s) in (\"\")"=w353) -> ("States Out"=w352:string)  [unwired: 14 in]
      }
      frame "---------- UI ----------" {
        # "Do not put any code in this frame.\n(It is a separator no-op. You can make a copy of this frame to create a new UI frame)"
        n131 = call <vilib>:"Add State(s) to Queue__JKI_lib_State_Machine.vi"("State(s) in (\"\")"=w358) -> ("States Out"=w357:string)  [unwired: 14 in]
      }
      frame "UI: Initialize" {
      }
      frame "UI: Cursor Set" {
        # "Argument"
        # "Set and Unset Cursor Busy.\n(Usage: \"UI: Cursor Set >> Busy|Idle\")"
        n132 = case shown="\"Idle\", Default" w364 {
          tunnel: w366 -> [w371 w373]
          tunnel: [w370 w372] -> w365
          frame "Idle", Default {
            n133 = call <vilib>:"Unset Busy.vi"("error in (no error)"=w371) -> ("error out"=w370:errorcluster)  [unwired: 10 in]
          }
          frame "Busy" {
            n134 = call <vilib>:"Set Busy.vi"("error in (no error)"=w373) -> ("error out"=w372:errorcluster)  [unwired: 9 in, 1 out]
          }
        }
        n135 = call <vilib>:"Add State(s) to Queue__JKI_lib_State_Machine.vi"("State(s) in (\"\")"=w369) -> ("States Out"=w368:string)  [unwired: 14 in]
      }
      frame "UI: Front Panel State" {
        # "Argument"
        # "Set Front Panel Open or Closed\n(Usage: \"UI: Front Panel State >> Open|Close\")"
        n136 = Unbundle By Name(w377) -> ("Core.Current VI Reference"=w376:refnum<vi>)
        n137 = case shown="\"Minimize\", \"Minimized\"" w375 {
          tunnel: w379 -> [w387 w402 w413 w426 w439]
          tunnel: [w389 w403 w415 w428 w441] -> w378
          tunnel: w376 -> [w388 w400 w414 w427 w440]
          frame "Open", "Standard", Default {
            w382 = T5."Standard" ("State")
            n138 = property class="VI"(reference=w388, error in=w387) -> (reference out=w385:refnum<vi>, error out=w386:errorcluster, "FP.State"=w384:T5)
            n139 = Not Equal?(x=w384, y=w382) -> (x != y?=w383:bool)
            n140 = case shown="True" w383 {
              tunnel: [w393 w395] -> w389
              tunnel: w386 -> [w392 w395]
              tunnel: w385 -> [w391 _]
              tunnel: w382 -> [w390 _]
              frame True {
                n141 = invoke class="VI" method="FP.Open"(reference=w391, error in=w392, "Activate"=TRUE, "State"=w390) -> (error out=w393:errorcluster)  [unwired: 1 in, 4 out]
              }
              frame False {
              }
            }
          }
          frame "Close", "Closed" {
            n142 = property class="VI"(reference=w400, error in=w402) -> (reference out=w399:refnum<vi>, error out=w401:errorcluster, "FP.State"=w397:T5)
            n143 = Not Equal?(x=w397, y=T5."Closed" ("Front Panel Window:State")) -> (x != y?=w396:bool)
            n144 = case shown="True" w396 {
              tunnel: [w404 w407] -> w403
              tunnel: w401 -> [w404 w406]
              tunnel: w399 -> [_ w405]
              frame False {
              }
              frame True {
                n145 = invoke class="VI" method="FP.Close"(reference=w405, error in=w406) -> (error out=w407:errorcluster)  [unwired: 1 in, 2 out]
              }
            }
          }
          frame "Hidden", "Hide" {
            w408 = T5."Hidden" ("State")
            n146 = property class="VI"(reference=w414, error in=w413) -> (reference out=w411:refnum<vi>, error out=w412:errorcluster, "FP.State"=w410:T5)
            n147 = Not Equal?(x=w410, y=w408) -> (x != y?=w409:bool)
            n148 = case shown="True" w409 {
              tunnel: [w419 w420] -> w415
              tunnel: w412 -> [w418 w420]
              tunnel: w411 -> [w417 _]
              tunnel: w408 -> [w416 _]
              frame True {
                n149 = invoke class="VI" method="FP.Open"(reference=w417, error in=w418, "State"=w416) -> (error out=w419:errorcluster)  [unwired: 2 in, 4 out]
              }
              frame False {
              }
            }
          }
          frame "Minimize", "Minimized" {
            w421 = T5."Minimized" ("State")
            n150 = property class="VI"(reference=w427, error in=w426) -> (reference out=w424:refnum<vi>, error out=w425:errorcluster, "FP.State"=w423:T5)
            n151 = Not Equal?(x=w423, y=w421) -> (x != y?=w422:bool)
            n152 = case shown="True" w422 {
              tunnel: [w432 w433] -> w428
              tunnel: w425 -> [w431 w433]
              tunnel: w424 -> [w430 _]
              tunnel: w421 -> [w429 _]
              frame True {
                n153 = invoke class="VI" method="FP.Open"(reference=w430, error in=w431, "State"=w429) -> (error out=w432:errorcluster)  [unwired: 2 in, 4 out]
              }
              frame False {
              }
            }
          }
          frame "Maximize", "Maximized" {
            w434 = T5."Maximized" ("State")
            n154 = property class="VI"(reference=w440, error in=w439) -> (reference out=w437:refnum<vi>, error out=w438:errorcluster, "FP.State"=w436:T5)
            n155 = Not Equal?(x=w436, y=w434) -> (x != y?=w435:bool)
            n156 = case shown="True" w435 {
              tunnel: [w445 w446] -> w441
              tunnel: w438 -> [w444 w446]
              tunnel: w437 -> [w443 _]
              tunnel: w434 -> [w442 _]
              frame True {
                n157 = invoke class="VI" method="FP.Open"(reference=w443, error in=w444, "State"=w442) -> (error out=w445:errorcluster)  [unwired: 2 in, 4 out]
              }
              frame False {
              }
            }
          }
        }
        n158 = call <vilib>:"Add State(s) to Queue__JKI_lib_State_Machine.vi"("State(s) in (\"\")"=w381) -> ("States Out"=w380:string)  [unwired: 14 in]
      }
      frame "---------- Macro ----------" {
        # "Do not put any code in this frame.\n(It is a separator no-op. You can make a copy of this frame to create a new Macro frame)"
        n159 = call <vilib>:"Add State(s) to Queue__JKI_lib_State_Machine.vi"("State(s) in (\"\")"=w451) -> ("States Out"=w450:string)  [unwired: 14 in]
      }
      frame "Macro: Initialize" {
        n160 = call <vilib>:"Add State(s) to Queue__JKI_lib_State_Machine.vi"("State(s) in Front (\"\")"="Data: Initialize\nInitialize Core Data\nEvents: Register\nUI: Initialize\n// UI: Front Panel State >> Open\n\n\nAction: Read Config\nAction: Update  TBL", "State(s) in (\"\")"=w457) -> ("States Out"=w456:string)  [unwired: 13 in]
      }
      frame "Macro: Update" {
        n161 = call <vilib>:"Add State(s) to Queue__JKI_lib_State_Machine.vi"("State(s) in Front (\"\")"="", "State(s) in (\"\")"=w463) -> ("States Out"=w462:string)  [unwired: 13 in]
      }
      frame "Macro: Exit" {
        # "Exit Macro\n(This is called once, when the VI exits)"
        n162 = Unbundle By Name(w472) -> ("Core.Close Panel on Exit?"=w471:bool)
        n163 = Select(t="UI: Front Panel State >> Close", s=w471, f="") -> (s? t:f=w468:string)
        n164 = call <vilib>:"Add State(s) to Queue__JKI_lib_State_Machine.vi"("State(s) in Front (\"\")"="Action: Write Config", "State(s) in (\"\")"=w468, "State(s) at Back (\"\")"="Data: Cleanup\nEvents: Unregister\nExit") -> ("States Out"=w466:string)  [unwired: 12 in]
        n165 = call <vilib>:"Add State(s) to Queue__JKI_lib_State_Machine.vi"("State(s) in Front (\"\")"=w466, "State(s) in (\"\")"=w475) -> ("States Out"=w474:string)  [unwired: 13 in]
      }
      frame "---------- Action ----------" {
      }
      frame "Action: Read Config" {
        n166 = disable-structure shown="Disabled" {
          disable-tunnel: [w496 w506] -> w486
          disable-tunnel: w485 -> [w495 _]
          disable-tunnel: [w493 _] -> w484
          disable-tunnel: w483 -> [w492 w506]
          disable-tunnel: [w489 _] -> w480
          frame Disabled {
            n167 = Unbundle By Name(w492) -> ("Alarm developer settings name"=w491, "Alarm customer settings name"=w490)
            n168 = call "Read ConfigInterface.vi"("GUI in"=w495) -> ("ConfigInterface"=w494:refnum<class "ConfigInterface.lvclass">)  [unwired: 9 in, 1 out]
            n169 = in-place {
              in-place-border: w494 -> [w497]
              in-place-border: [w503] -> w493
              in-place-border: w491 -> [w502]
              in-place-border: w490 -> [w501]
              in-place-border: [w498] -> w489
              n170 = in-place-cluster #4(w492) -> ("GUI Alarm developer settings"=w505, "GUI Alarm customer settings"=w500)
              n171 = call "ReadOrCreate.vim"("reference in"=w497, "Type and Defaults"=w500, "Name"=w501) -> ("Data"=w499:T10, "error out"=w498:errorcluster)  [unwired: 8 in, 3 out]
              n172 = call "ReadOrCreate.vim"("reference in"=w497, "Type and Defaults"=w505, "Name"=w502) -> ("Data"=w504:T11, "error out"=w503:errorcluster)  [unwired: 8 in, 3 out]
              n173 = in-place-cluster #4("GUI Alarm developer settings"=w504, "GUI Alarm customer settings"=w499) -> (w496:T7)
            }
          }
          frame Enabled {
          }
        }
        n174 = Merge Errors(w484, w480, w481) -> (w482:errorcluster)
      }
      frame "Action: Write Config" {
        n175 = disable-structure shown="Disabled" {
          disable-tunnel: w510 -> [w523 _]
          disable-tunnel: w509 -> [w521 _]
          disable-tunnel: w508 -> [w520 _]
          disable-tunnel: [w515 _] -> w507
          frame Disabled {
            n176 = Unbundle By Name(w520) -> ("GUI Alarm customer settings"=w513, "Alarm customer settings name"=w514, "GUI Alarm developer settings"=w518, "Alarm developer settings name"=w519)
            n177 = call "Read ConfigInterface.vi"("GUI in"=w523) -> ("ConfigInterface"=w522:refnum<class "ConfigInterface.lvclass">)  [unwired: 9 in, 1 out]
            n178 = call-dynamic "Write.vi"("reference in"=w522, "Data"=w518, "Name"=w519, "error in (no error)"=w521) -> ("reference out"=w516:refnum<class "ConfigInterface.lvclass">, "error out"=w517:errorcluster)  [unwired: 8 in, 2 out]
            n179 = call-dynamic "Write.vi"("reference in"=w516, "Data"=w513, "Name"=w514, "error in (no error)"=w517) -> ("error out"=w515:errorcluster)  [unwired: 8 in, 3 out]
          }
          frame Enabled {
          }
        }
      }
      frame "Action: Update  TBL" {
        n180 = Unbundle By Name(w538) -> ("Steps ref"=w537:refnum<vi>, "Curr Script"=w526:T2)
        n181 = Unbundle By Name(w526) -> ("Steps"=w530:T3[])
        n182 = call "Script to Tbl.vi"("Script"=w526) -> ("Tbl"=w536:string[][])  [unwired: 14 in]
        n183 = call "Script to Graph.vi"("Script"=w526, "tr"=1.0) -> ("XY Data"=→"XY Graph - Dark":cluster{"X":dbl[], "Y":dbl[]}[])  [unwired: 13 in]
        n184 = property class="MCListbox (strict)"(reference=w537, error in=w535, "ItemNames"=w536) -> (reference out=w527:refnum<vi>, error out=w534:errorcluster, "Value"=w533:i32)
        n185 = Array Size(array=w530) -> (size(s)=w529:i32)
        n186 = call "range.vi"("size"=w529, "index"=w533) -> ("lower limit"=w528:i32)  [unwired: 13 in]
        n187 = Index Array(array=w530, index=w528) -> (element=w532:T3)
        n188 = property class="MCListbox (strict)"(reference=w527, "Value"=w528) -> ()  [unwired: 1 in, 2 out]
        n189 = call "RT to GUI Step.vi"("STEP"=w532) -> ("GUI Step"=w531:T1)  [unwired: 14 in]
        n190 = local write "GUI Step"(w531) -> ()
      }
    }
  }
  "error out" <- w6
